vi "ExSubGrabOneFrame.vi"(4 "Display Title":string, 5 "error in":errorcluster, 6 "ROI Cluster":T1={"X Start"=1, "X End"=1, "X Bin/Group"=1, "Y Start"=1, "Y End"=1, "Y Bin/Group"=1} {"Y Bin/Group" min=1 max=4096 step=1; "Y End" min=1 max=10000 step=1; "Y Start" min=1 max=10000 step=1; "X Bin/Group" min=1 max=4096 step=1; "X End" min=1 max=10000 step=1; "X Start" min=1 max=10000 step=1}, 7 "Exposure":dbl format="%.2f", 8 "Camera Handle":u32) -> (0 "error out":errorcluster, 1 "Image Handle":u32, 2 "Display Handle":u32, 3 "Camera Handle out":u32)   [LabVIEW 2010]
panel:
  # "ExSubGrabOneFrame:\nThis is a sub vi that given an ROI cluster,\nan exposure, and a title; colllects one \nframe  and displays it.\nThis sub-vi collects in Async mode so \nshould be valid for any camera."
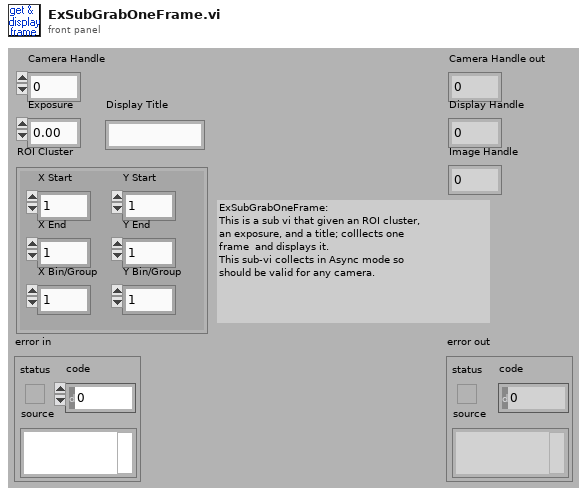
[diagram p1: front panel]
types:
  T1 = cluster{"X Start":u32, "X End":u32, "X Bin/Group":u32, "Y Start":u32, "Y End":u32, "Y Bin/Group":u32}
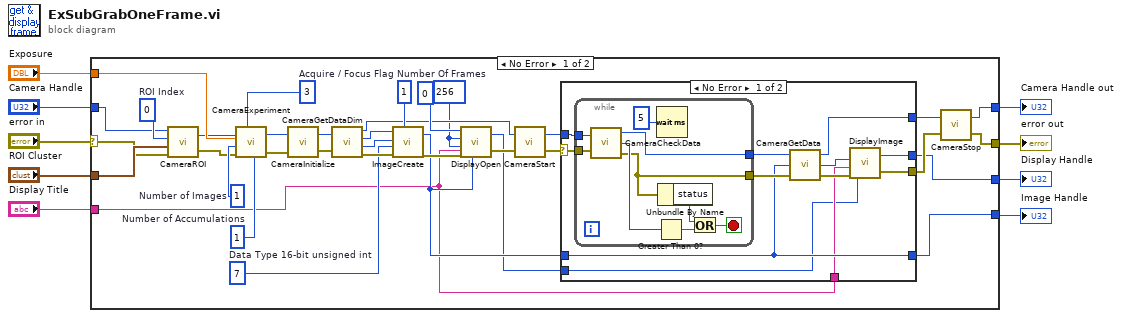
[diagram p0: block diagram]
diagram:
  n1 = case shown="No Error" "error in" {
    selector: "error in" -> [w21 w71]
    tunnel: "Camera Handle" -> [w20 w72]
    tunnel: [w36 w72] -> w8
    tunnel: "ROI Cluster" -> [w35 _]
    tunnel: "Display Title" -> [w25 _]
    tunnel: [w14 w71] -> w5
    tunnel: "Exposure" -> [w23 _]
    tunnel: [w22 w70] -> w2
    tunnel: [w15 w70] -> w1
    frame No Error {
      w12 = 256
      w31 = 7  # Data Type 16-bit unsigned int
      w37 = u32 0  # ROI Index
      w38 = u32 3  # Acquire / Focus Flag
      w34 = u32 1  # Number Of Frames
      w39 = u32 1  # Number of Images
      w40 = u32 1  # Number of Accumulations
      n2 = call <userlib>:"CameraROI.vi"("error in"=w21, "ROI Params"=w35, "ROI Index"=w37, "Camera Handle"=w20) -> ("error out"=w18:errorcluster, "Camera Handle"=w19:u32)
      n3 = call <userlib>:"CameraExperiment.vi"("Number of Accumulations"=w40, "Acquire / Focus Flag"=w38, "error in"=w18, "Number of Images"=w39, "Exposure (sec)"=w23, "Camera Handle"=w19) -> ("error out"=w16:errorcluster, "Camera Handle"=w17:u32)
      n4 = call <userlib>:"CameraInitialize.vi"("error in"=w16, "Camera Handle"=w17) -> ("error out"=w42:errorcluster, "Camera Handle"=w41:u32)
      n5 = call <userlib>:"CameraGetDataDim.vi"("Camera Handle"=w41, "error in"=w42) -> ("Camera Handle"=w28:u32, "Xdim"=w11:u32, "Ydim"=w10:u32, "error out"=w33:errorcluster)
      n6 = call <userlib>:"ImageCreate.vi"("X dimension"=w11, "Y dimension"=w10, "Data Type"=w31, "error in"=w33, "Number Of Frames"=w34) -> ("Image Handle"=w27:u32, "error out"=w32:errorcluster)
      n7 = call <userlib>:"DisplayOpen.vi"("Display Title"=w25, "Image Handle"=w27, "error in"=w32, "Display Height"=w12, "Display Width"=w12, "Display Type"=0) -> ("error out"=w29:errorcluster, "Display Handle"=w26:u32)
      n8 = call <userlib>:"CameraStart.vi"("error in"=w29, "Camera Handle"=w28) -> ("error out"=w13:errorcluster, "Camera Handle"=w43:u32)
      n9 = case shown="No Error" w13 {
        selector: w13 -> [w51 w69]
        tunnel: w27 -> [w52 w67]
        tunnel: w43 -> [w56 w68]
        tunnel: [w50 w69] -> w24
        tunnel: [w53 w68] -> w44
        tunnel: [w52 w67] -> w15
        tunnel: w26 -> [w46 w66]
        tunnel: w25 -> [w47 _]
        tunnel: [w45 w66] -> w22
        frame No Error {
          n10 = while {
            tunnel: w56 -> [w65]
            tunnel: [w62] -> w54
            tunnel: [w63] -> w55
            tunnel: w51 -> [w57]
            stop <- w59 stop-if-true
            n11 = call <userlib>:"CameraCheckData.vi"("Camera Handle"=w65, "error in"=w57) -> ("Camera Handle"=w63:u32, "Number Of Frames Available"=w64:i32, "error out"=w62:errorcluster)
            n12 = Greater Than 0?(x=w64) -> (x > 0?=w60:bool)
            n13 = Wait (ms)(milliseconds to wait=u32 5) -> ()  [unwired: 1 out]
            n14 = Unbundle By Name(w62) -> ("status"=w61:bool)
            n15 = Or(x=w61, y=w60) -> (x .or. y?=w59:bool)
          }
          n16 = call <userlib>:"CameraGetData.vi"("error in"=w54, "Data Handle"=w52, "Camera Handle"=w55) -> ("error out"=w48:errorcluster, "Data Handle"=w49:u32, "Camera Handle"=w53:u32)
          n17 = call <userlib>:"DisplayImage.vi"("error in"=w48, "Title"=w47, "Image Handle"=w49, "Display Handle"=w46) -> ("error out"=w50:errorcluster, "Display Handle"=w45:u32)
        }
        frame Error {
        }
      }
      n18 = call <userlib>:"CameraStop.vi"("error in"=w24, "Camera Handle"=w44) -> ("error out"=w14:errorcluster, "Camera Handle"=w36:u32)
    }
    frame Error {
      w70 = 0
    }
  }
  "Camera Handle out" <- w8
  "Display Handle" <- w2
  "error out" <- w5
  "Image Handle" <- w1
